vi "opencvSegmentLL2.vi"(5 "allocate size":i32=10000, 7 "allocate":bool=TRUE, 10 "threshold":sgl=600.0, 11 "ImgIn":u16[][](array[numeric])) -> (2 "NeuronN":u16, 3 "NeuronYX":u16[][](array[numeric]))   [LabVIEW 2017]
uses:
  dll/wormUtilities/x64/Release/wormUtilities.dll
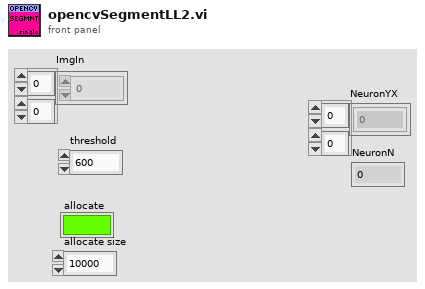
[diagram p1: front panel]
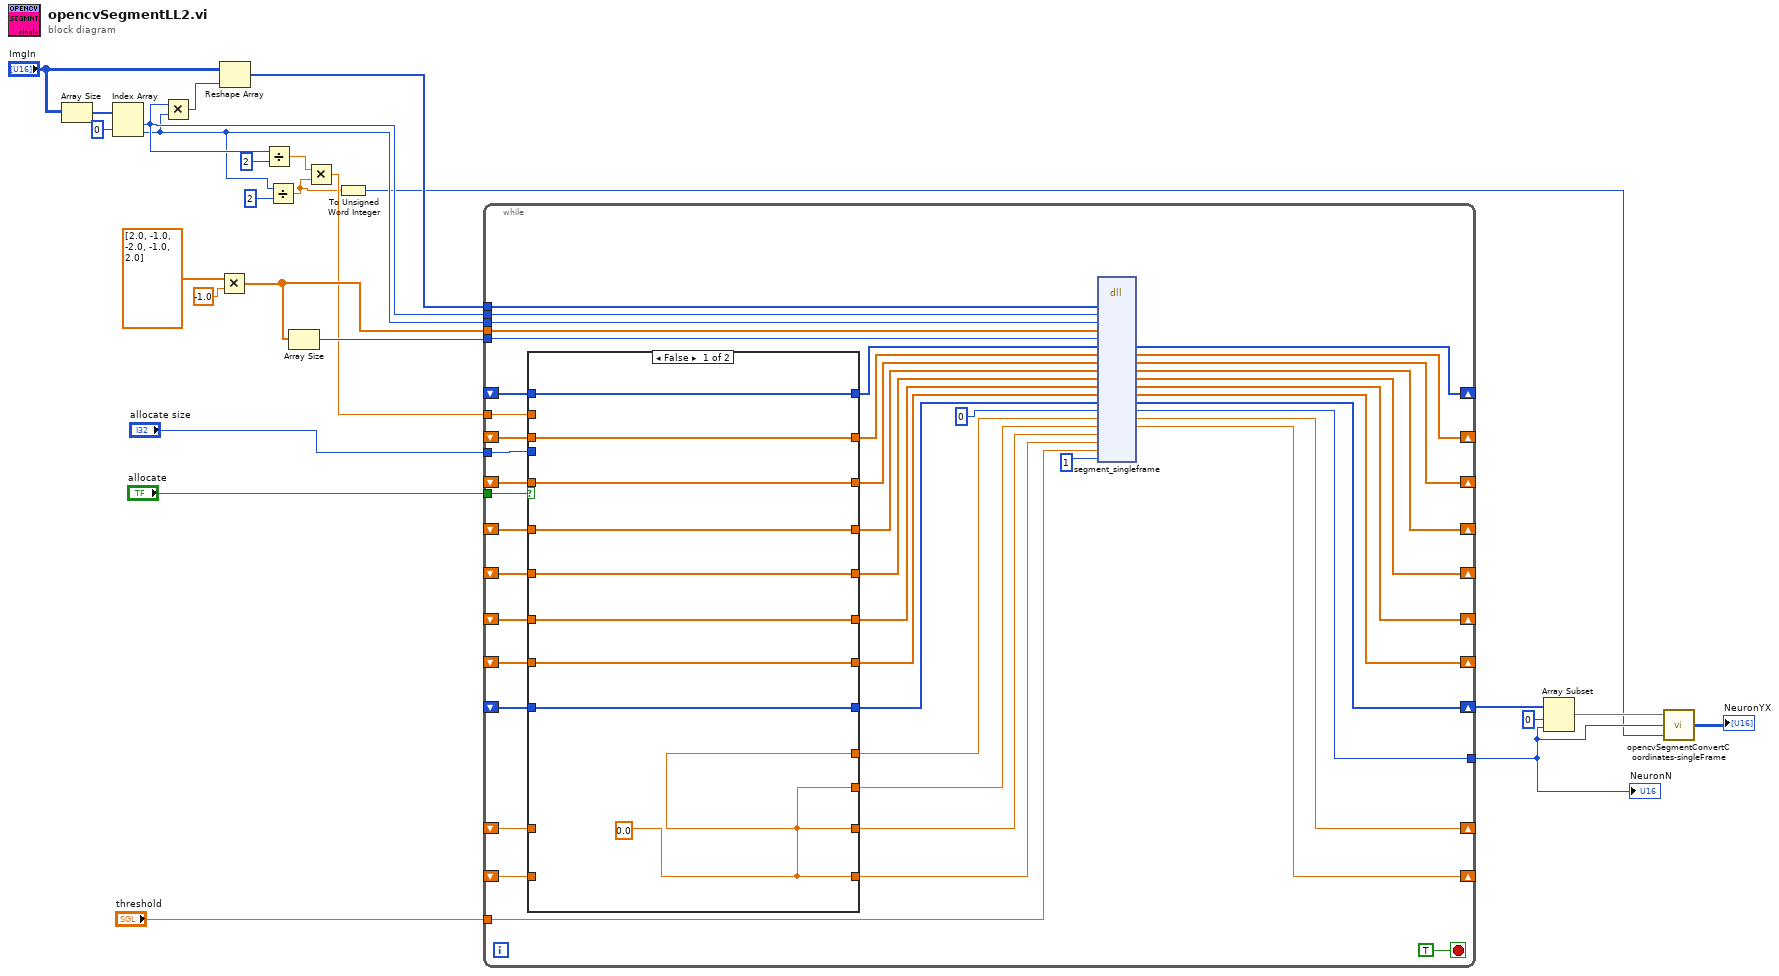
[diagram p0: block diagram]
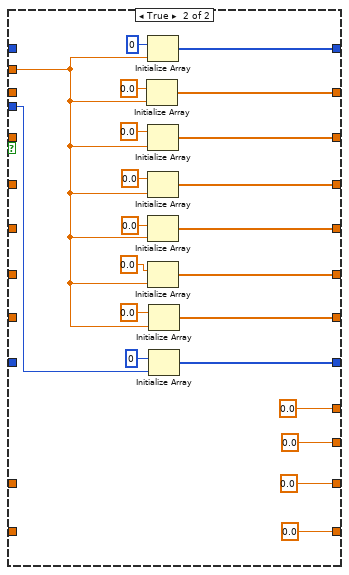
[diagram p2: hidden frame]
diagram:
  n1 = Array Size(array="ImgIn") -> (size(s)=w21:i32[])
  n2 = Index Array(array=w21, index #1=0 ("index")) -> (element #1=w11:i32, element #2=w8:i32)  [unwired: 1 in]
  n3 = Multiply(x=w11, y=w8) -> (x*y=w19:i32)
  n4 = Multiply(x=sgl[] [2.0, -1.0, -2.0, -1.0, 2.0], y=sgl -1.0) -> (x*y=w23:sgl[])
  n5 = Reshape Array("ImgIn", w19) -> (w17:u16[])
  n6 = Divide(x=w11, y=2) -> (x/y=w7:dbl)
  n7 = Divide(x=w8, y=2) -> (x/y=w3:dbl)
  n8 = Array Size(array=w23) -> (size(s)=w22:i32)
  n9 = Multiply(x=w7, y=w3) -> (x*y=w6:dbl)
  n10 = To Unsigned Word Integer(number=w3) -> (unsigned 16bit integer=w2:u16)
  n11 = while {
    tunnel: w23 -> [w70]
    tunnel: w22 -> [w69]
    tunnel: w8 -> [w67]
    tunnel: w11 -> [w66]
    tunnel: w17 -> [w65]
    tunnel: "allocate" -> [w64]
    tunnel: "allocate size" -> [w63]
    tunnel: "threshold" -> [w54]
    shift-right: [w53] -> _
    shift-left: _ -> [w52]
    shift-right: [w51] -> _
    shift-left: _ -> [w50]
    shift-right: [w49] -> _
    shift-left: _ -> [w48]
    shift-right: [w47] -> _
    shift-left: _ -> [w46]
    shift-right: [w45] -> _
    shift-left: _ -> [w44]
    shift-right: [w43] -> _
    shift-left: _ -> [w42]
    shift-right: [w41] -> _
    shift-left: _ -> [w40]
    shift-right: [w39] -> w13
    shift-left: _ -> [w38]
    tunnel: [w37] -> w4
    shift-right: [w34] -> _
    shift-left: _ -> [w30]
    shift-right: [w35] -> _
    shift-left: _ -> [w31]
    tunnel: w6 -> [w28]
    stop <- TRUE stop-if-true
    n12 = case shown="False" w64 {
      tunnel: w63 -> [_ w83]
      tunnel: [w79 w96] -> w62
      tunnel: [w78 w95] -> w61
      tunnel: [w77 w94] -> w60
      tunnel: [w76 w93] -> w59
      tunnel: [w75 w89] -> w58
      tunnel: [w74 w88] -> w57
      tunnel: [w73 w87] -> w56
      tunnel: [w72 w86] -> w55
      tunnel: w52 -> [w79 _]
      tunnel: w50 -> [w78 _]
      tunnel: w48 -> [w77 _]
      tunnel: w46 -> [w76 _]
      tunnel: w44 -> [w75 _]
      tunnel: w42 -> [w74 _]
      tunnel: w40 -> [w73 _]
      tunnel: w38 -> [w72 _]
      tunnel: [w71 0.0] -> w33
      tunnel: [w71 0.0] -> w32
      tunnel: w31 -> [_ _]
      tunnel: w30 -> [_ _]
      tunnel: w28 -> [_ w82]
      tunnel: [w71 0.0 ("maxBXY")] -> w27
      tunnel: [w71 0.0 ("maxBXY")] -> w26
      frame False {
        w71 = 0.0
      }
      frame True {
        n13 = Initialize Array(sgl 0.0 ("element"), w82) -> (w95:sgl[])
        n14 = Initialize Array(u16 0 ("element"), w82) -> (w96:u16[])
        n15 = Initialize Array(sgl 0.0 ("element"), w82) -> (w94:sgl[])
        n16 = Initialize Array(sgl 0.0 ("element"), w82) -> (w93:sgl[])
        n17 = Initialize Array(sgl 0.0 ("element"), w82) -> (w89:sgl[])
        n18 = Initialize Array(sgl 0.0 ("element"), w82) -> (w88:sgl[])
        n19 = Initialize Array(sgl 0.0 ("element"), w82) -> (w87:sgl[])
        n20 = Initialize Array(u16 0 ("element"), w83) -> (w86:u16[])
      }
    }
    n21 = dll-call lib="C:/Users/francesco/dev/pump-probe/dll/wormUtilities/x64/Release/wormUtilities.dll" fn="segment_singleframe"("ImgIn"=w65, "sizex"=w66, "sizey"=w67, "arrC"=w70, "sizeC"=w69, "ArrA"=w62, "ArrB"=w61, "ArrBX"=w60, "ArrBY"=w59, "ArrBth"=w58, "ArrBdil"=w57, "ArrUno"=w56, "NeuronXY"=w55, "NeuronN"=u16 0, "maxX"=w26, "maxY"=w27, "maxXInStack"=w33, "maxYInStack"=w32, "threshold"=w54, "resize"=i8 1) -> ("ArrA"=w53:u16[], "ArrB"=w51:sgl[], "ArrBX"=w49:sgl[], "ArrBY"=w47:sgl[], "ArrBth"=w45:sgl[], "ArrBdil"=w43:sgl[], "ArrUno"=w41:sgl[], "NeuronXY"=w39:u16[], "NeuronN"=w37:u16, "maxX"=w35:dbl, "maxY"=w34:dbl)  [unwired: 13 in, 2 out]
  }
  "NeuronN" <- w4
  n22 = Array Subset(array=w13, index=0, length=w4) -> (w5:u16[])
  n23 = call "opencvSegmentConvertCoordinates-singleFrame.vi"("sizex2"=w2, "NeuronN"=w4, "NeuronXY"=w5) -> ("XY"=→"NeuronYX":u16[][])
